vi "test-trajectory-transform-ALL.vi"(8 "error in (no error)":errorcluster) -> (0 "error out 2":errorcluster, 3 "Test Passed":bool)   [LabVIEW 2019]
panel:
  out "TEst 1":bool
  out "Test 2":bool
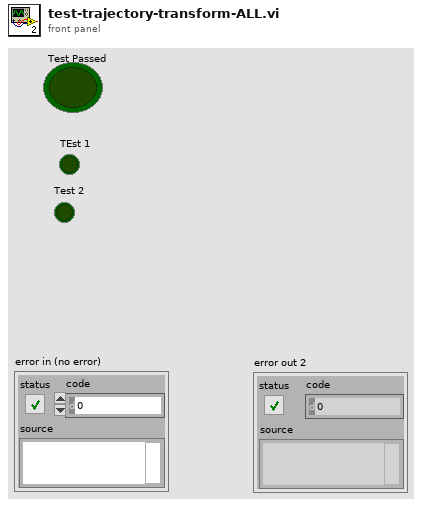
[diagram p1: front panel]
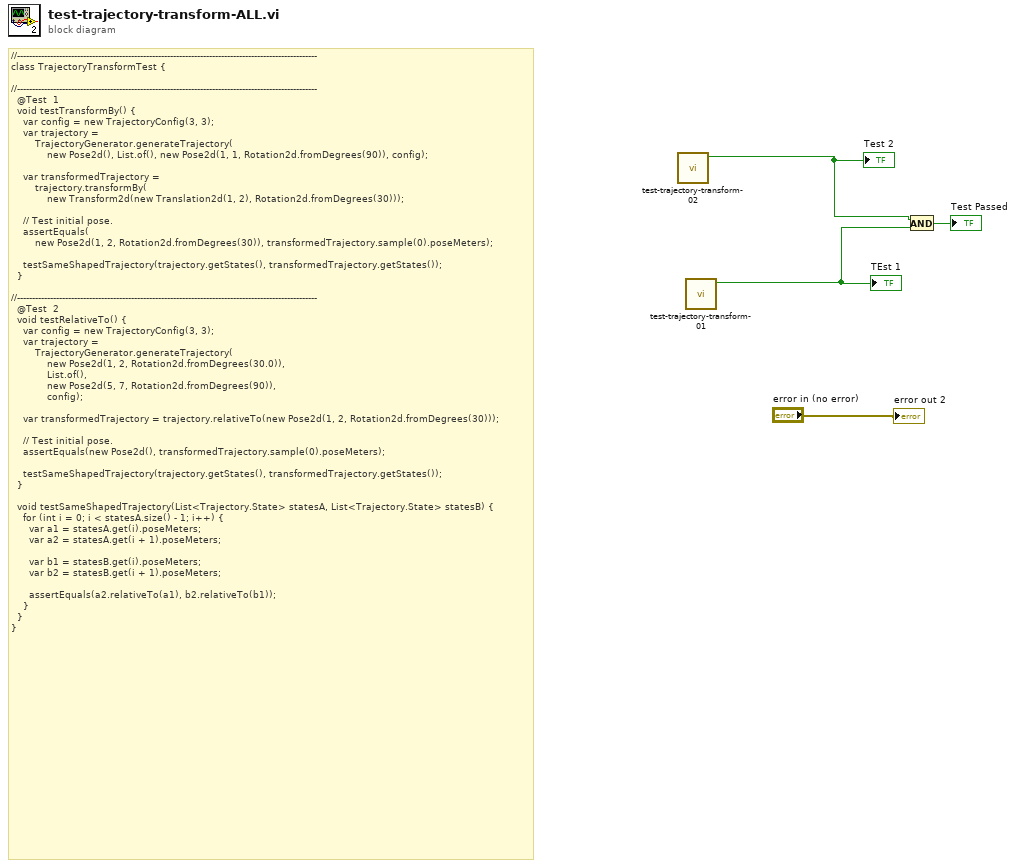
[diagram p0: block diagram]
diagram:
  # "//----------------------------------------------------------------------------------------------------\nclass TrajectoryTransformTest {\n\n//----------------------------------------------------------------------------------------------------\n  @Test  1\n  void testTransformBy() {\n    var config = new TrajectoryConfig(3, 3);\n    var trajectory =\n        TrajectoryGenerator.generateTrajectory(\n            new Pose2d(), List.of(), new Pose2d(1, 1, Rotation2d.fromDegrees(90)), config);\n\n    var transformedTrajectory =\n        trajectory.transformBy(\n            new Transform2d(new Translation2d(1, 2), Rotation2d.fromDegrees(30)));\n\n    // Test initial pose.\n    assertEquals(\n        new Pose2d(1, 2, Rotation2d.fromDegrees(30)), transformedTrajectory.sample(0).poseMeters);\n\n    testSameShapedTrajectory(trajectory.getStates(), transformedTrajectory.getStates());\n  }\n\n//----------------------------------------------------------------------------------------------------\n  @Test  2\n  void testRelativeTo() {\n    var config = new TrajectoryConfig(3, 3);\n    var trajectory =\n        TrajectoryGenerator.generateTrajectory(\n            new Pose2d(1, 2, Rotation2d.fromDegrees(30.0)),\n            List.of(),\n            new Pose2d(5, 7, Rotation2d.fromDegrees(90)),\n            config);\n\n    var transformedTrajectory = trajectory.relativeTo(new Pose2d(1, 2, Rotation2d.fromDegrees(30)));\n\n    // Test initial pose.\n    assertEquals(new Pose2d(), transformedTrajectory.sample(0).poseMeters);\n\n    testSameShapedTrajectory(trajectory.getStates(), transformedTrajectory.getStates());\n  }\n\n  void testSameShapedTrajectory(List<Trajectory.State> statesA, List<Trajectory.State> statesB) {\n    for (int i = 0; i < statesA.size() - 1; i++) {\n      var a1 = statesA.get(i).poseMeters;\n      var a2 = statesA.get(i + 1).poseMeters;\n\n      var b1 = statesB.get(i).poseMeters;\n      var b2 = statesB.get(i + 1).poseMeters;\n\n      assertEquals(a2.relativeTo(a1), b2.relativeTo(b1));\n    }\n  }\n}"
  n1 = call "test-trajectory-transform-02.vi"() -> ("Test Passed"=w2:bool)  [unwired: 11 in]
  "Test 2" <- w2
  n2 = call "test-trajectory-transform-01.vi"() -> ("Test Passed"=w3:bool)  [unwired: 11 in]
  "TEst 1" <- w3
  n3 = And(x=w2, y=w3) -> (x .and. y?=→"Test Passed":bool)
  "error out 2" <- "error in (no error)"
